vi "Example 4.vi"() -> ()   [LabVIEW 2018, in "LcWebView.lvclass"]
uses:
  LcWebView.lvclass
  C:/Projects/LcWebView2/LcWebView/LcWebView_class/data/Microsoft.Web.WebView2.WinForms.dll
  data/Microsoft.Web.WebView2.WinForms.dll
panel:
  in  "Web":refnum<k24>(container)
  out "Error Out":errorcluster
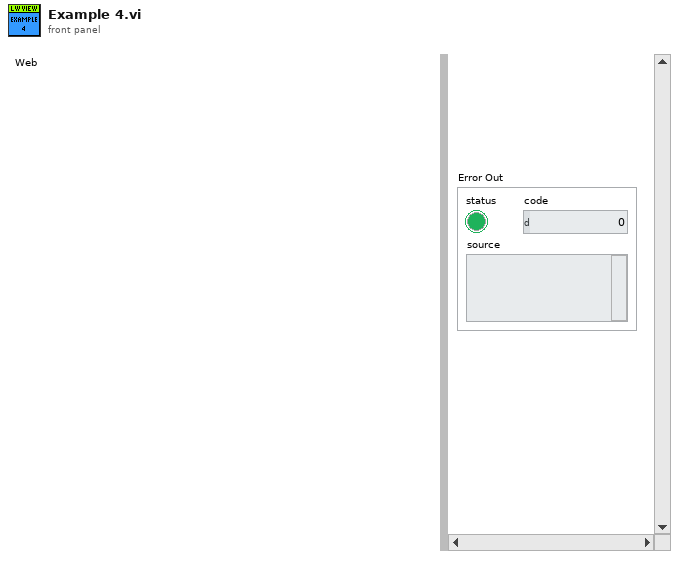
[diagram p1: front panel]
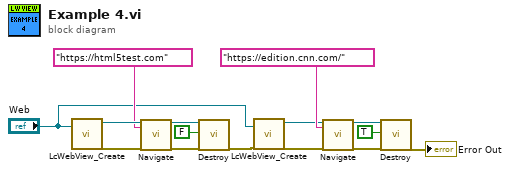
[diagram p0: block diagram]
diagram:
  n1 = call "LcWebView_Create.vi"("Webview container"="Web") -> ("reference out"=w15:refnum<class "LcWebView.lvclass">, "Error Out"=w14:errorcluster)  [unwired: 11 in, 6 out]
  n2 = call-dynamic "Navigate.vi"("reference in"=w15, "URL"="https://html5test.com", "Error In"=w14) -> ("reference out"=w12:refnum<class "LcWebView.lvclass">, "Error Out"=w11:errorcluster)  [unwired: 14 in, 1 out]
  n3 = call-dynamic "Destroy.vi"("reference in"=w12, "BlankBrowser(True)"=FALSE, "Error In"=w11) -> ("Error Out"=w5:errorcluster)  [unwired: 15 in, 1 out]
  n4 = call "LcWebView_Create.vi"("Webview container"="Web", "Error In"=w5) -> ("reference out"=w6:refnum<class "LcWebView.lvclass">, "Error Out"=w7:errorcluster)  [unwired: 10 in, 6 out]
  n5 = call-dynamic "Navigate.vi"("reference in"=w6, "URL"="https://edition.cnn.com/", "Error In"=w7) -> ("reference out"=w9:refnum<class "LcWebView.lvclass">, "Error Out"=w10:errorcluster)  [unwired: 14 in, 1 out]
  n6 = call-dynamic "Destroy.vi"("reference in"=w9, "BlankBrowser(True)"=TRUE, "Error In"=w10) -> ("Error Out"=→"Error Out":errorcluster)  [unwired: 15 in, 1 out]
